vi "Arm.vi"(4 "Request type":T1=enum."User command", 6 "Init work":bool, 7 "Update period":dbl, 8 "error in (no error)":errorcluster, 9 "Last request":bool, 10 "Requester":string, 11 "Lockin Digitizer in":refnum<class "Lockin Digitizer.lvclass">) -> (0 "error out":errorcluster, 3 "Lockin Digitizer out":refnum<class "Lockin Digitizer.lvclass">)   [LabVIEW 2021, in "Lockin Digitizer.lvclass"]
uses:
  Lockin Digitizer.lvclass
  Controllers/Process Controller/Request type.ctl
  NHMFL_Core/Libraries/Instruments/Pulse Driver/Lockin Digitizer Driver/Lockin Digitizer Driver.lvclass
  C:/GitHub/NHMFL_Core/Libraries/Instruments/Pulse Driver/Pulse Driver.lvclass
  Lockin Digitizer.lvclass/Lockin Digitizer.ctl
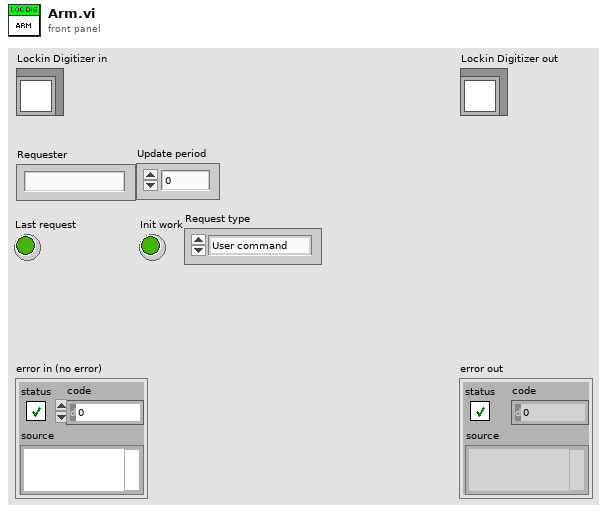
[diagram p1: front panel]
types:
  T1 = typedef "Request type.ctl" = enum16{"Process complete", "User command", "Auto-restart", "Error"}
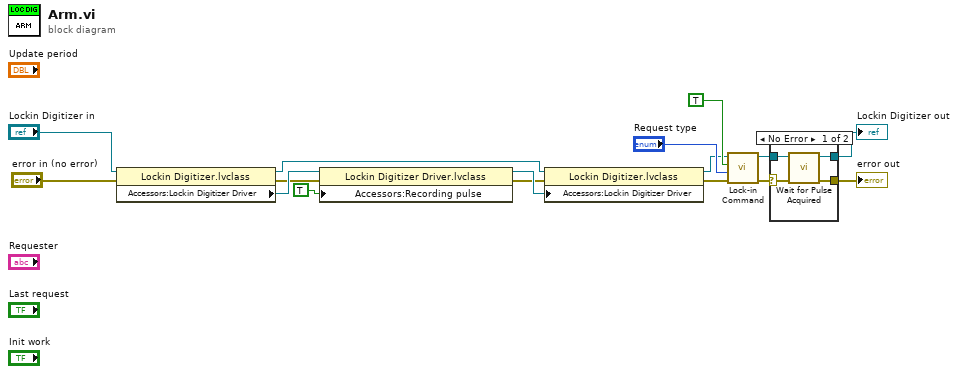
[diagram p0: block diagram]
diagram:
  n1 = property class="Lockin Digitizer.lvclass"(reference="Lockin Digitizer in", error in="error in (no error)") -> (reference out=w4:refnum<class "Lockin Digitizer.lvclass">, error out=w8:errorcluster, "Accessors:Lockin Digitizer Driver"=w10:refnum<class "Lockin Digitizer Driver.lvclass">)
  n2 = property class="Lockin Digitizer Driver.lvclass"(reference=w10, error in=w8, "Accessors:Recording pulse"=TRUE ("Recording pulse")) -> (reference out=w7:refnum<class "Lockin Digitizer Driver.lvclass">, error out=w6:errorcluster)
  n3 = property class="Lockin Digitizer.lvclass"(reference=w4, error in=w6, "Accessors:Lockin Digitizer Driver"=w7) -> (reference out=w3:refnum<class "Lockin Digitizer.lvclass">, error out=w5:errorcluster)
  n4 = call-dynamic "Lock-in Command.vi"("error in (no error)"=w5, "Request type"="Request type", "Lock-in"=TRUE, "Lockin Digitizer in"=w3) -> ("error out"=w1:errorcluster, "Lockin Digitizer out"=w2:refnum<class "Lockin Digitizer.lvclass">)  [unwired: 5 in, 1 out]
  n5 = case shown="No Error" w1 {
    selector: w1 -> [w20 w21]
    tunnel: w2 -> [w19 w22]
    tunnel: [w18 w22] -> w14
    tunnel: [w17 w21] -> w13
    frame No Error {
      n6 = call-dynamic "Wait for Pulse Acquired.vi"("error in (no error)"=w20, "Pulse Recorder Actor in"=w19) -> ("error out"=w17:errorcluster, "Pulse Recorder Actor out"=w18:refnum<class "Lockin Digitizer.lvclass">)  [unwired: 8 in]
    }
    frame Error {
    }
  }
  "error out" <- w13
  "Lockin Digitizer out" <- w14
